vi "DCON-Read.vi"(0 "VRN in":refnum<visa-resource-name>, 11 "error in (no error)":errorcluster) -> (4 "VRN Dup":refnum<visa-resource-name>, 6 "DataCluster":T1, 10 "Boolean array":bool[](array[boolean]), 15 "error out":errorcluster)   [LabVIEW 2011]
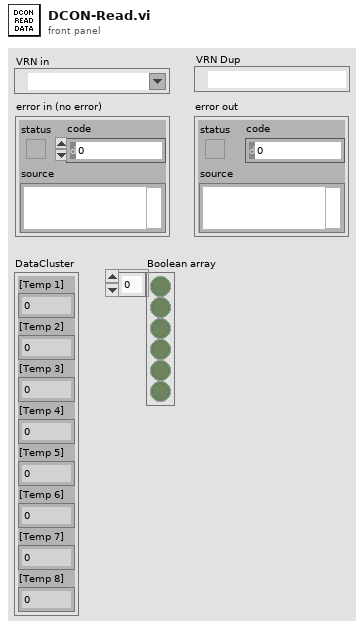
[diagram p1: front panel]
types:
  T1 = cluster{"[Temp 1]":dbl, "[Temp 2]":dbl, "[Temp 3]":dbl, "[Temp 4]":dbl, "[Temp 5]":dbl, "[Temp 6]":dbl, "[Temp 7]":dbl, "[Temp 8]":dbl}
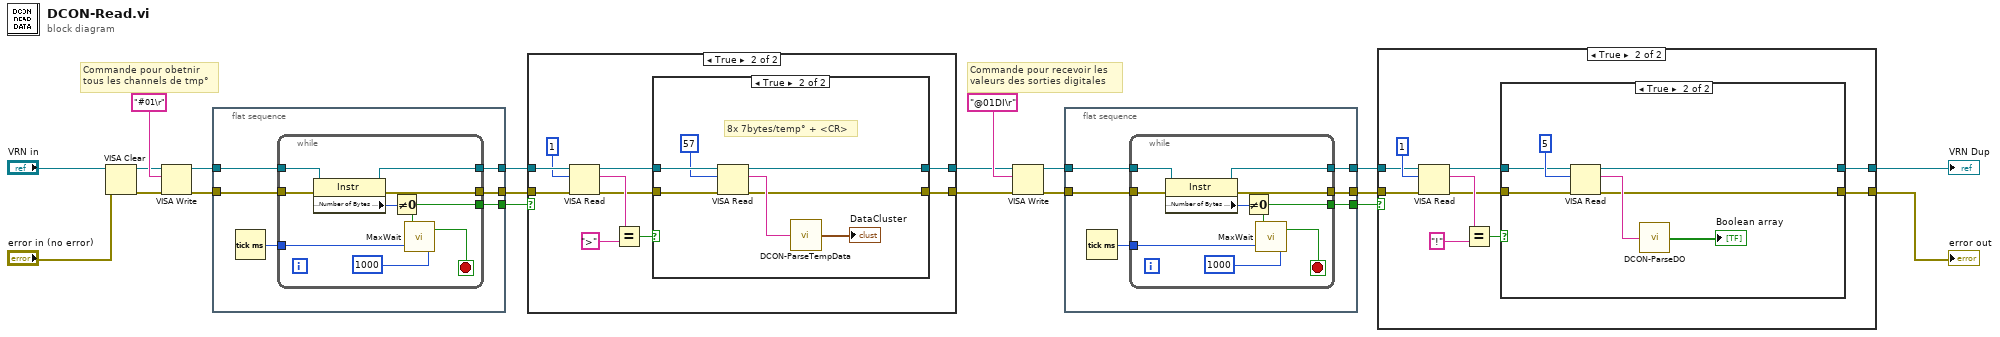
[diagram p0: block diagram]
diagram:
  # "Commande pour recevoir les\nvaleurs des sorties digitales"
  # "Commande pour obetnir\ntous les channels de tmp°"
  n1 = VISA Clear(VISA resource name="VRN in", error in (no error)="error in (no error)") -> (VISA resource name out=w17:refnum<visa-resource-name>, error out=w16:errorcluster)
  n2 = VISA Write(VISA resource name=w17, write buffer="#01\r", error in (no error)=w16) -> (VISA resource name out=w19:refnum<visa-resource-name>, error out=w18:errorcluster)  [unwired: 1 out]
  n3 = flat-sequence {
    tunnel: w19 -> [w26]
    tunnel: w18 -> [w25]
    tunnel: [w23] -> w12
    tunnel: [w22] -> w11
    tunnel: [w21] -> w13
    frame #0 {
      n4 = Tick Count (ms)() -> (millisecond timer value=w24:u32)
      n5 = while {
        tunnel: w26 -> [w31]
        tunnel: w25 -> [w32]
        tunnel: w24 -> [w34]
        tunnel: [w30] -> w22
        tunnel: [w29] -> w23
        tunnel: [w27] -> w21
        stop <- w35 stop-if-true
        n6 = property class="Instr"(reference=w31, error in=w32) -> (reference out=w30:refnum<visa-resource-name>, error out=w29:errorcluster, "Serial Settings:Number of Bytes at Serial Port"=w28:u32)
        n7 = Not Equal To 0?(x=w28) -> (x != 0?=w27:bool)
        n8 = call "MaxWait.vi"("WaitLimit (ms)"=u32 1000, "StartTick (from outside the node)"=w34, "Valeur entrante"=w27) -> ("break ?"=w35:bool)
      }
    }
  }
  n9 = case shown="True" w13 {
    tunnel: w12 -> [w36 w46]
    tunnel: w11 -> [w37 w47]
    tunnel: [w36 w39] -> w6
    tunnel: [w37 w38] -> w7
    frame False {
    }
    frame True {
      n10 = VISA Read(VISA resource name=w47, byte count=u32 1, error in (no error)=w46) -> (VISA resource name out=w41:refnum<visa-resource-name>, read buffer=w44:string, error out=w40:errorcluster)  [unwired: 1 out]
      n11 = Equal?(x=w44, y=">") -> (x = y?=w42:bool)
      n12 = case shown="True" w42 {
        tunnel: w41 -> [w49 w56]
        tunnel: w40 -> [w48 w55]
        tunnel: [w49 w51] -> w38
        tunnel: [w48 w50] -> w39
        frame False {
          # "Commande non comprise ..."
        }
        frame True {
          # "8x 7bytes/temp° + <CR>"
          n13 = VISA Read(VISA resource name=w56, byte count=u32 57, error in (no error)=w55) -> (VISA resource name out=w51:refnum<visa-resource-name>, read buffer=w53:string, error out=w50:errorcluster)  [unwired: 1 out]
          n14 = call "DCON-ParseTempData.vi"("Read Buffer"=w53) -> ("DataCluster"=→"DataCluster":T1)  [unwired: 14 in]
        }
      }
    }
  }
  n15 = VISA Write(VISA resource name=w7, write buffer="@01DI\r", error in (no error)=w6) -> (VISA resource name out=w9:refnum<visa-resource-name>, error out=w10:errorcluster)  [unwired: 1 out]
  n16 = flat-sequence {
    tunnel: w9 -> [w62]
    tunnel: w10 -> [w61]
    tunnel: [w59] -> w4
    tunnel: [w58] -> w3
    tunnel: [w57] -> w5
    frame #0 {
      n17 = Tick Count (ms)() -> (millisecond timer value=w60:u32)
      n18 = while {
        tunnel: w62 -> [w67]
        tunnel: w61 -> [w68]
        tunnel: w60 -> [w70]
        tunnel: [w66] -> w58
        tunnel: [w65] -> w59
        tunnel: [w63] -> w57
        stop <- w71 stop-if-true
        n19 = property class="Instr"(reference=w67, error in=w68) -> (reference out=w66:refnum<visa-resource-name>, error out=w65:errorcluster, "Serial Settings:Number of Bytes at Serial Port"=w64:u32)
        n20 = Not Equal To 0?(x=w64) -> (x != 0?=w63:bool)
        n21 = call "MaxWait.vi"("WaitLimit (ms)"=u32 1000, "StartTick (from outside the node)"=w70, "Valeur entrante"=w63) -> ("break ?"=w71:bool)
      }
    }
  }
  n22 = case shown="True" w5 {
    tunnel: w4 -> [w72 w80]
    tunnel: w3 -> [w73 w79]
    tunnel: [w73 w75] -> w2
    tunnel: [w72 w74] -> w1
    frame False {
    }
    frame True {
      n23 = VISA Read(VISA resource name=w79, byte count=u32 1, error in (no error)=w80) -> (VISA resource name out=w76:refnum<visa-resource-name>, read buffer=w82:string, error out=w77:errorcluster)  [unwired: 1 out]
      n24 = Equal?(x=w82, y="!") -> (x = y?=w78:bool)
      n25 = case shown="True" w78 {
        tunnel: w77 -> [w84 w90]
        tunnel: w76 -> [w85 w91]
        tunnel: [w85 w87] -> w75
        tunnel: [w84 w86] -> w74
        frame False {
        }
        frame True {
          n26 = VISA Read(VISA resource name=w91, byte count=u32 5, error in (no error)=w90) -> (VISA resource name out=w87:refnum<visa-resource-name>, read buffer=w89:string, error out=w86:errorcluster)  [unwired: 1 out]
          n27 = call "DCON-ParseDO.vi"("Read Buffer"=w89) -> ("Boolean array"=→"Boolean array":bool[])  [unwired: 14 in]
        }
      }
    }
  }
  "error out" <- w1
  "VRN Dup" <- w2
